vi "ClearValues.vi"(8 "error in (no error)":errorcluster, 11 "history in":variant) -> (0 "error out":errorcluster, 3 "history out":variant)   [LabVIEW 2017, in "TestPanel.lvlib"]
uses:
  <vilib>/addons/InsightCM/Devices/Shared/Common/TestPanel/TestPanel.lvlib
  <vilib>/addons/InsightCM/MessageBus/Base/controls/TestPanelTimeSeries.ctl
  <vilib>/addons/InsightCM/MessageBus/Base/controls/TestPanelValue.ctl
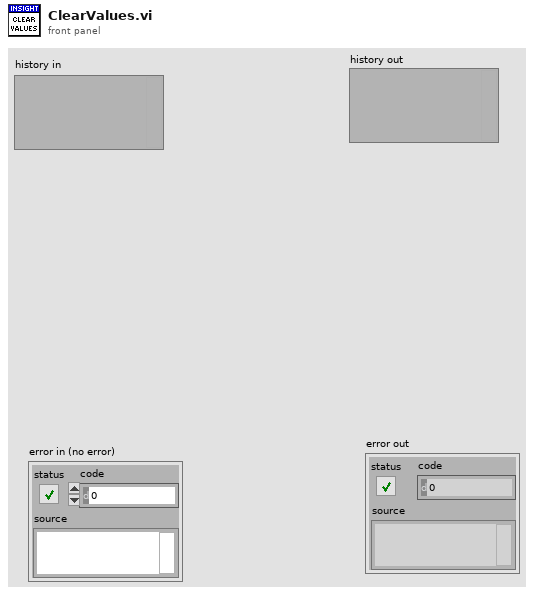
[diagram p1: front panel]
types:
  T1 = typedef "TestPanelTimeSeries.ctl" = cluster{"TrendPointId":string, "AssetName":string, "MetricName":string, "Unit":string, "Values":T2[]}
  T2 = typedef "TestPanelValue.ctl" = cluster{"Value":dbl, "Timestamp":i64, "Invalid":bool}
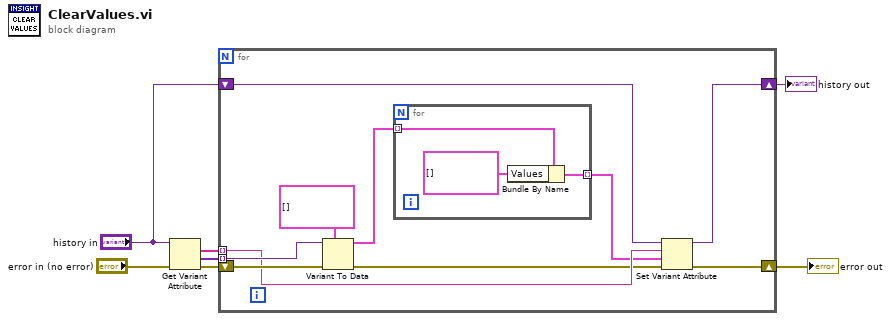
[diagram p0: block diagram]
diagram:
  n1 = Get Variant Attribute(Variant="history in", error in="error in (no error)") -> (names=w5:string[], values=w6:variant[], error out=w7:errorcluster)  [unwired: 2 in, 1 out]
  n2 = for {
    shift-right: [w11] -> w3
    shift-left: w7 -> [w16]
    tunnel: w6 -> [w15] mode=indexing
    tunnel: w5 -> [w13] mode=indexing
    shift-right: [w8] -> w1
    shift-left: "history in" -> [w10]
    n3 = Variant To Data(error in=w16, type=T1[] [], Variant=w15) -> (data=w14:T1[], error out=w12:errorcluster)
    n4 = for {
      tunnel: w14 -> [w20] mode=indexing
      tunnel: [w18] -> w9 mode=indexing
      n5 = Bundle By Name(cluster=w20, "Values"=T2[] []) -> (w18:T1)
    }
    n6 = Set Variant Attribute(Variant=w10, name=w13, value=w9, error in=w12) -> (Variant out=w8:variant, error out=w11:errorcluster)  [unwired: 1 out]
  }
  "error out" <- w3
  "history out" <- w1
